vi "format_EIS_data.vi"() -> ()   [LabVIEW 2014]
uses:
  <vilib>/Utility/file.llb/Read From Spreadsheet File (string).vi
  <vilib>/Utility/file.llb/Write To Spreadsheet File (string).vi
panel:
  in  "how data should be formatted after running this program":string[][](table)
  in  "Path of file":path
  out "number of data rows":string
  # "1. Select a .txt file saved from a nyquist plot in the Zahner software\n2. Click run. Formatted file will be saved in same location with name \n    \"x_formatted\", where \"x\" is original file name"
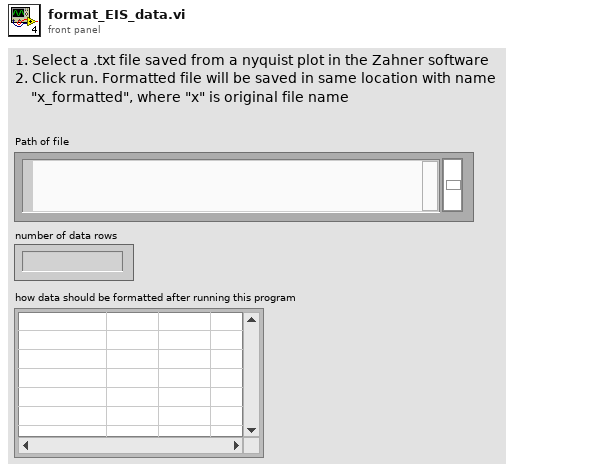
[diagram p1: front panel]
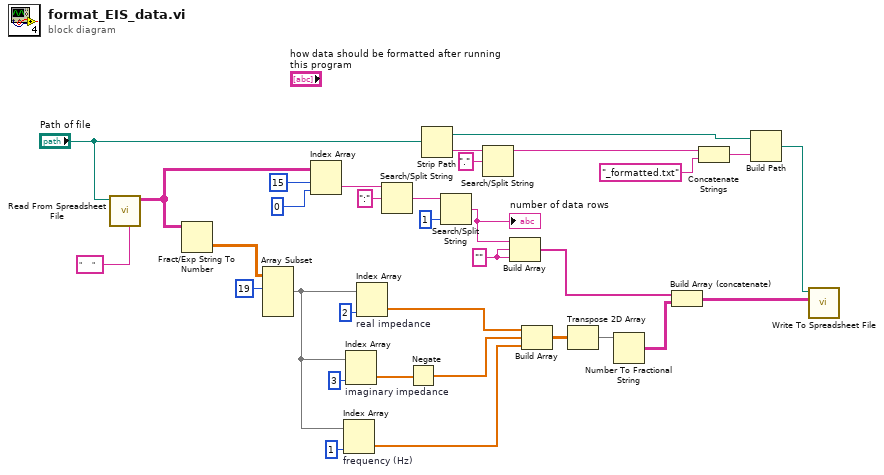
[diagram p0: block diagram]
diagram:
  w24 = "" ("delimiter (\\t)")
  n1 = call-poly <vilib>:"Read From Spreadsheet File.vi"("delimiter (\\t)"="     " ("delimiter (\\t)"), "file path (dialog if empty)"="Path of file") -> ("all rows"=w20:string[][])  [unwired: 5 in, 4 out]
  n2 = Fract/Exp String To Number(string=w20) -> (number=w19:dbl[][])  [unwired: 3 in, 1 out]
  n3 = Array Subset(array=w19, index (row)=19 ("index")) -> (w16:dbl[][])  [unwired: 3 in]
  n4 = Index Array ("number of data rows")(array=w20, index (row)=15, index (col)=0 ("disabled index (col)")) -> (element=w29:string)
  n5 = Index Array "frequency (Hz)"(array=w16, index (col)=1 ("index (row)")) -> (element=w18:dbl[])  [unwired: 1 in]
  n6 = Index Array "imaginary impedance"(array=w16, index (col)=3 ("index (row)")) -> (element=w14:dbl[])  [unwired: 1 in]
  n7 = Index Array "real impedance"(array=w16, index (col)=2 ("index (row)")) -> (element=w15:dbl[])  [unwired: 1 in]
  n8 = Search/Split String(string=w29, search string/char (-)=":") -> (match + rest of string=w28:string)  [unwired: 1 in, 2 out]
  n9 = Negate(x=w14) -> (-x=w13:dbl[])
  n10 = Strip Path(path="Path of file") -> (stripped path=w7:path, name=w3:string)
  n11 = Search/Split String(string=w28, offset (0)=1) -> (match + rest of string=w25:string)  [unwired: 1 in, 2 out]
  "number of data rows" <- w25
  n12 = Search/Split String(string=w3, search string/char (-)=".") -> (substring before match=w2:string)  [unwired: 1 in, 2 out]
  n13 = Build Array(w25, w24, w24) -> (w23:string[])
  n14 = Build Array(w15, w13, w18) -> (w12:dbl[][])
  n15 = Transpose 2D Array(2D array=w12) -> (transposed array=w11:dbl[][])
  n16 = Number To Fractional String(number=w11) -> (F-format string=w10:string[][])  [unwired: 3 in]
  n17 = Build Array (concatenate)(w23, w10) -> (w9:string[][])
  n18 = Concatenate Strings(w2, "_formatted.txt" ("string")) -> (w6:string)
  n19 = Build Path(base path=w7, name or relative path=w6) -> (appended path=w5:path)
  n20 = call-poly <vilib>:"Write To Spreadsheet File.vi"("2D data"=w9, "file path (dialog if empty)"=w5) -> ()  [unwired: 6 in, 1 out]
